vi "runtest parse settings.vi"(11 "POST (empty)":T1) -> (0 "SeqCount":i32, 1 "Hide System Fields?":bool, 2 "Quickmode?":bool, 3 "Run Step":i32)   [LabVIEW 2011]
uses:
  Addons/internet/utils/keyedarr.llb/Keyed Array.ctl
  Addons/internet/utils/strutil.llb/Case Matching.ctl
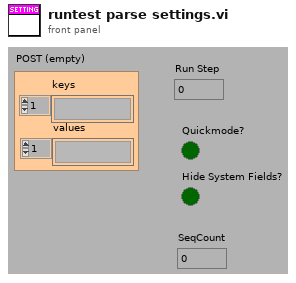
[diagram p1: front panel]
types:
  T1 = typedef "Keyed Array.ctl" = cluster{"keys":string[], "values":string[]}
  T2 = typedef "Case Matching.ctl" = enum16{"a != A", "a == A", "system"}
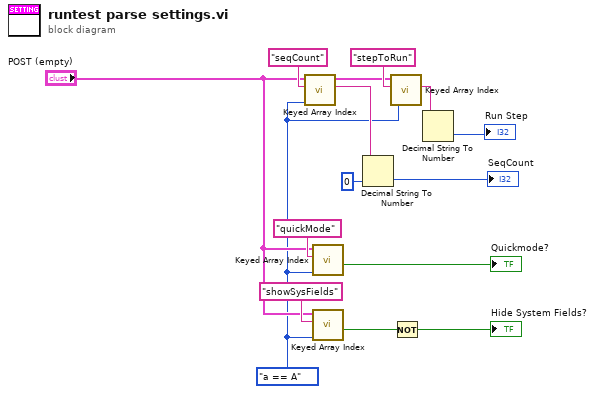
[diagram p0: block diagram]
diagram:
  w6 = Case_Matching."a == A" ("case matching (sensitive)")
  n1 = call "Keyed Array Index.vi"("case matching (sensitive)"=w6, "key"="seqCount", "array in"="POST (empty)") -> ("value"=w10:string, "duplicate array"=w9:T1)  [unwired: 1 in, 2 out]
  n2 = call "Keyed Array Index.vi"("case matching (sensitive)"=w6, "key"="quickMode", "array in"="POST (empty)") -> ("valid key"=→"Quickmode?":bool)  [unwired: 1 in, 3 out]
  n3 = call "Keyed Array Index.vi"("case matching (sensitive)"=w6, "key"="showSysFields", "array in"="POST (empty)") -> ("valid key"=w3:bool)  [unwired: 1 in, 3 out]
  n4 = Decimal String To Number(string=w10, default (0L)=0 ("default (0 I32)")) -> (number=→"SeqCount":i32)  [unwired: 2 out]
  n5 = call "Keyed Array Index.vi"("case matching (sensitive)"=w6, "key"="stepToRun", "array in"=w9) -> ("value"=w11:string)  [unwired: 1 in, 3 out]
  n6 = Not(x=w3) -> (.not. x?=→"Hide System Fields?":bool)
  n7 = Decimal String To Number(string=w11) -> (number=→"Run Step":i32)  [unwired: 3 out]
